vi "Interpolation_Solver.vi"(2 "Points Between":i32=10 min=0 step=1, 3 "Type of Interpolation":T2(ring), 4 "Data":dbl[][](array[numeric])=[[0.0, 1.0], [1.0, 2.700000047683716], [2.0, 7.400000095367432], [3.0, 150.0], [4.0, 80.0], [5.0, 220.0]] format="%.2f") -> (0 "Interpolated Data":dbl[](array[numeric])=[0.0, 0.09090909090909091, 0.18181818181818182, 0.2727272727272727, 0.36363636363636365, 0.45454545454545453, 0.5454545454545454, 0.6363636363636364, 0.7272727272727273, 0.8181818181818182, 0.9090909090909091, 1.0, 1.0909090909090908, 1.1818181818181819, 1.2727272727272727, 1.3636363636363635, 1.4545454545454546, 1.5454545454545454, 1.6363636363636365, 1.7272727272727273, 1.8181818181818181, 1.9090909090909092, 2.0, 2.090909090909091, 2.1818181818181817, 2.272727272727273, 2.3636363636363638, 2.4545454545454546, 2.5454545454545454, 2.6363636363636362, 2.727272727272727, 2.8181818181818183, 2.909090909090909, 3.0, 3.090909090909091, 3.1818181818181817, 3.272727272727273, 3.3636363636363638, 3.4545454545454546, 3.5454545454545454, 3.6363636363636362, 3.727272727272727, 3.8181818181818183, 3.909090909090909, 4.0, 4.090909090909091, 4.181818181818182, 4.2727272727272725, 4.363636363636363, 4.454545454545454, 4.545454545454546, 4.636363636363637, 4.7272727272727275, 4.818181818181818, 4.909090909090909, 5.0] format="%.2f", 1 "Interpolated X Axis":dbl[](array[numeric])=[0.0, 0.16666666666666666, 0.3333333333333333, 0.5, 0.6666666666666666, 0.8333333333333334, 1.0, 1.1666666666666667, 1.3333333333333333, 1.5, 1.6666666666666667, 1.8333333333333333, 2.0, 2.1666666666666665, 2.3333333333333335, 2.5, 2.6666666666666665, 2.8333333333333335, 3.0, 3.1666666666666665, 3.3333333333333335, 3.5, 3.6666666666666665, 3.8333333333333335, 4.0, 4.166666666666667, 4.333333333333333, 4.5, 4.666666666666667, 4.833333333333333, 5.0, 5.166666666666667, 5.333333333333333, 5.5, 5.666666666666667, 5.833333333333333, 6.0, 6.166666666666667, 6.333333333333333, 6.5, 6.666666666666667, 6.833333333333333, 7.0, 7.166666666666667, 7.333333333333333, 7.5, 7.666666666666667, 7.833333333333333, 8.0, 8.166666666666666, 8.333333333333334, 8.5, 8.666666666666666, 8.833333333333334, 9.0, 9.166666666666666, 9.333333333333334, 9.5, 9.666666666666666, 9.833333333333334, 10.0, 10.166666666666666, 10.333333333333334, 10.5, 10.666666666666666, 10.833333333333334, 11.0, 11.166666666666666, 11.333333333333334, 11.5, 11.666666666666666, 11.833333333333334, 12.0, 12.166666666666666, 12.333333333333334, 12.5, 12.666666666666666, 12.833333333333334, 13.0, 13.166666666666666, 13.333333333333334, 13.5, 13.666666666666666, 13.833333333333334, 14.0, 14.166666666666666, 14.333333333333334, 14.5, 14.666666666666666, 14.833333333333334, 15.0, 15.166666666666666, 15.333333333333334, 15.5, 15.666666666666666, 15.833333333333334, 16.0, 16.166666666666668, 16.333333333333332, 16.5, 16.666666666666668, 16.833333333333332, 17.0, 17.166666666666668, 17.333333333333332, 17.5, 17.666666666666668, 17.833333333333332, 18.0, 18.166666666666668, 18.333333333333332, 18.5, 18.666666666666668, 18.833333333333332, 19.0, 19.166666666666668, 19.333333333333332, 19.5, 19.666666666666668, 19.833333333333332, 20.0, 20.166666666666668, 20.333333333333332, 20.5, 20.666666666666668, 20.833333333333332, 21.0, 21.166666666666668, 21.333333333333332, 21.5, 21.666666666666668, 21.833333333333332, 22.0, 22.166666666666668, 22.333333333333332, 22.5, 22.666666666666668, 22.833333333333332, 23.0, 23.166666666666668, 23.333333333333332, 23.5, 23.666666666666668, 23.833333333333332, 24.0, 24.166666666666668, 24.333333333333332, 24.5, 24.666666666666668, 24.833333333333332, 25.0, 25.166666666666668, 25.333333333333332, 25.5, 25.666666666666668, 25.833333333333332, 26.0, 26.166666666666668, 26.333333333333332, 26.5, 26.666666666666668, 26.833333333333332, 27.0, 27.166666666666668, 27.333333333333332, 27.5, 27.666666666666668, 27.833333333333332, 28.0, 28.166666666666668, 28.333333333333332, 28.5, 28.666666666666668, 28.833333333333332, 29.0, 29.166666666666668, 29.333333333333332, 29.5, 29.666666666666668, 29.833333333333332, 30.0, 30.166666666666668, 30.333333333333332, 30.5, 30.666666666666668, 30.833333333333332, 31.0, 31.166666666666668, 31.333333333333332, 31.5, 31.666666666666668, 31.833333333333332, 32.0, 32.166666666666664, 32.333333333333336, 32.5, 32.666666666666664, 32.833333333333336, 33.0, 33.166666666666664, 33.333333333333336, 33.5, 33.666666666666664, 33.833333333333336, 34.0, 34.166666666666664, 34.333333333333336, 34.5, 34.666666666666664, 34.833333333333336, 35.0, 35.166666666666664, 35.333333333333336, 35.5, 35.666666666666664, 35.833333333333336, 36.0, 36.166666666666664, 36.333333333333336, 36.5, 36.666666666666664, 36.833333333333336, 37.0, 37.166666666666664, 37.333333333333336, 37.5, 37.666666666666664, 37.833333333333336, 38.0, 38.166666666666664, 38.333333333333336, 38.5, 38.666666666666664, 38.833333333333336, 39.0, 39.166666666666664, 39.333333333333336, 39.5, 39.666666666666664, 39.833333333333336, 40.0, 40.166666666666664, 40.333333333333336, 40.5, 40.666666666666664, 40.833333333333336, 41.0, 41.166666666666664, 41.333333333333336, 41.5, 41.666666666666664, 41.833333333333336, 42.0, 42.166666666666664, 42.333333333333336, 42.5, 42.666666666666664, 42.833333333333336, 43.0, 43.166666666666664, 43.333333333333336, 43.5, 43.666666666666664, 43.833333333333336, 44.0, 44.166666666666664, 44.333333333333336, 44.5, 44.666666666666664, 44.833333333333336, 45.0, 45.166666666666664, 45.333333333333336, 45.5, 45.666666666666664, 45.833333333333336, 46.0, 46.166666666666664, 46.333333333333336, 46.5, 46.666666666666664, 46.833333333333336, 47.0, 47.166666666666664, 47.333333333333336, 47.5, 47.666666666666664, 47.833333333333336, 48.0, 48.166666666666664, 48.333333333333336, 48.5, 48.666666666666664, 48.833333333333336, 49.0, 49.166666666666664, 49.333333333333336, 49.5, 49.666666666666664, 49.833333333333336, 50.0, 50.166666666666664, 50.333333333333336, 50.5, 50.666666666666664, 50.833333333333336, 51.0, 51.166666666666664, 51.333333333333336, 51.5, 51.666666666666664, 51.833333333333336, 52.0, 52.166666666666664, 52.333333333333336, 52.5, 52.666666666666664, 52.833333333333336, 53.0, 53.166666666666664, 53.333333333333336, 53.5, 53.666666666666664, 53.833333333333336, 54.0, 54.166666666666664, 54.333333333333336, 54.5, 54.666666666666664, 54.833333333333336, 55.0, 55.166666666666664, 55.333333333333336, 55.5, 55.666666666666664, 55.833333333333336, 56.0, 56.166666666666664, 56.333333333333336, 56.5, 56.666666666666664, 56.833333333333336, 57.0, 57.166666666666664, 57.333333333333336, 57.5, 57.666666666666664, 57.833333333333336, 58.0, 58.166666666666664, 58.333333333333336, 58.5, 58.666666666666664, 58.833333333333336, 59.0, 59.166666666666664, 59.333333333333336, 59.5, 59.666666666666664, 59.833333333333336, 60.0, 60.166666666666664, 60.333333333333336, 60.5, 60.666666666666664, 60.833333333333336, 61.0, 61.166666666666664, 61.333333333333336, 61.5, 61.666666666666664, 61.833333333333336, 62.0, 62.166666666666664, 62.333333333333336, 62.5, 62.666666666666664, 62.833333333333336, 63.0, 63.166666666666664, 63.333333333333336, 63.5, 63.666666666666664, 63.833333333333336, 64.0, 64.16666666666667, 64.33333333333333, 64.5, 64.66666666666667, 64.83333333333333, 65.0, 65.16666666666667, 65.33333333333333, 65.5, 65.66666666666667, 65.83333333333333, 66.0, 66.16666666666667, 66.33333333333333, 66.5, 66.66666666666667, 66.83333333333333, 67.0, 67.16666666666667, 67.33333333333333, 67.5, 67.66666666666667, 67.83333333333333, 68.0, 68.16666666666667, 68.33333333333333, 68.5, 68.66666666666667, 68.83333333333333, 69.0, 69.16666666666667, 69.33333333333333, 69.5, 69.66666666666667, 69.83333333333333, 70.0, 70.16666666666667, 70.33333333333333, 70.5, 70.66666666666667, 70.83333333333333, 71.0, 71.16666666666667, 71.33333333333333, 71.5, 71.66666666666667, 71.83333333333333, 72.0, 72.16666666666667, 72.33333333333333, 72.5, 72.66666666666667, 72.83333333333333, 73.0, 73.16666666666667, 73.33333333333333, 73.5, 73.66666666666667, 73.83333333333333, 74.0, 74.16666666666667, 74.33333333333333, 74.5, 74.66666666666667, 74.83333333333333, 75.0, 75.16666666666667, 75.33333333333333, 75.5, 75.66666666666667, 75.83333333333333, 76.0, 76.16666666666667, 76.33333333333333, 76.5, 76.66666666666667, 76.83333333333333, 77.0, 77.16666666666667, 77.33333333333333, 77.5, 77.66666666666667, 77.83333333333333, 78.0, 78.16666666666667, 78.33333333333333, 78.5, 78.66666666666667, 78.83333333333333, 79.0, 79.16666666666667, 79.33333333333333, 79.5, 79.66666666666667, 79.83333333333333, 80.0, 80.16666666666667, 80.33333333333333, 80.5, 80.66666666666667, 80.83333333333333, 81.0, 81.16666666666667, 81.33333333333333, 81.5, 81.66666666666667, 81.83333333333333, 82.0, 82.16666666666667, 82.33333333333333, 82.5, 82.66666666666667, 82.83333333333333, 83.0, 83.16666666666667, 83.33333333333333, 83.5, 83.66666666666667, 83.83333333333333, 84.0, 84.16666666666667, 84.33333333333333, 84.5, 84.66666666666667, 84.83333333333333, 85.0, 85.16666666666667, 85.33333333333333, 85.5, 85.66666666666667, 85.83333333333333, 86.0, 86.16666666666667, 86.33333333333333, 86.5, 86.66666666666667, 86.83333333333333, 87.0, 87.16666666666667, 87.33333333333333, 87.5, 87.66666666666667, 87.83333333333333, 88.0, 88.16666666666667, 88.33333333333333, 88.5, 88.66666666666667, 88.83333333333333, 89.0, 89.16666666666667, 89.33333333333333, 89.5, 89.66666666666667, 89.83333333333333, 90.0, 90.16666666666667, 90.33333333333333, 90.5, 90.66666666666667, 90.83333333333333, 91.0, 91.16666666666667, 91.33333333333333, 91.5, 91.66666666666667, 91.83333333333333, 92.0, 92.16666666666667, 92.33333333333333, 92.5, 92.66666666666667, 92.83333333333333, 93.0, 93.16666666666667, 93.33333333333333, 93.5, 93.66666666666667, 93.83333333333333, 94.0, 94.16666666666667, 94.33333333333333, 94.5, 94.66666666666667, 94.83333333333333, 95.0, 95.16666666666667, 95.33333333333333, 95.5, 95.66666666666667, 95.83333333333333, 96.0, 96.16666666666667, 96.33333333333333, 96.5, 96.66666666666667, 96.83333333333333, 97.0, 97.16666666666667, 97.33333333333333, 97.5, 97.66666666666667, 97.83333333333333, 98.0, 98.16666666666667, 98.33333333333333, 98.5, 98.66666666666667, 98.83333333333333, 99.0, 99.16666666666667, 99.33333333333333, 99.5, 99.66666666666667, 99.83333333333333, 100.0, 100.16666666666667, 100.33333333333333, 100.5, 100.66666666666667, 100.83333333333333, 101.0, 101.16666666666667, 101.33333333333333, 101.5, 101.66666666666667, 101.83333333333333, 102.0, 102.16666666666667, 102.33333333333333] format="%.4f")   [LabVIEW 2019]
doc: "This example demonstrates the use of various interpolation VIs including:\n Linear Interpolation\n Polynomial Interpolation\n Spline Interpolation\n Rational Interpolation"
uses:
  <vilib>/Utility/file.llb/Read From Spreadsheet File (DBL).vi
  <vilib>/Utility/file.llb/Write To Spreadsheet File (DBL).vi
  <vilib>/Analysis/NI_AALPro.lvlib
panel:
  in  "data selector":T1(ring)
  out "Raw Data and Interpolated Data":cluster{dbl[], "Best Exponential Fit":dbl[]}[](graph)=[{[0.0, 1.0, 2.0, 3.0, 4.0, 5.0], "Best Exponential Fit"=[1.0, 2.700000047683716, 7.400000095367432, 150.0, 80.0, 220.0]}, {[0.0, 0.09090909090909091, 0.18181818181818182, 0.2727272727272727, 0.36363636363636365, 0.45454545454545453, 0.5454545454545454, 0.6363636363636364, 0.7272727272727273, 0.8181818181818182, 0.9090909090909091, 1.0, 1.0909090909090908, 1.1818181818181819, 1.2727272727272727, 1.3636363636363635, 1.4545454545454546, 1.5454545454545454, 1.6363636363636365, 1.7272727272727273, 1.8181818181818181, 1.9090909090909092, 2.0, 2.090909090909091, 2.1818181818181817, 2.272727272727273, 2.3636363636363638, 2.4545454545454546, 2.5454545454545454, 2.6363636363636362, 2.727272727272727, 2.8181818181818183, 2.909090909090909, 3.0, 3.090909090909091, 3.1818181818181817, 3.272727272727273, 3.3636363636363638, 3.4545454545454546, 3.5454545454545454, 3.6363636363636362, 3.727272727272727, 3.8181818181818183, 3.909090909090909, 4.0, 4.090909090909091, 4.181818181818182, 4.2727272727272725, 4.363636363636363, 4.454545454545454, 4.545454545454546, 4.636363636363637, 4.7272727272727275, 4.818181818181818, 4.909090909090909, 5.0], "Best Exponential Fit"=[1.0, 1.2152761356490307, 1.780613923204889, 2.575277433580718, 3.4785307376896637, 4.36963790644487, 5.127863010759482, 5.632470121546648, 5.762723309719508, 5.397886646191209, 4.417224201874898, 2.700000047683716, 0.20566834793003874, -2.785556359476875, -5.91326944322851, -8.817066272016389, -11.136542214532014, -12.511292639466877, -12.580912915512496, -10.98499841136037, -7.363144495702005, -1.3549465372288942, 7.400000095367432, 19.083237862020354, 33.16086053716275, 48.92009972385246, 65.64818702514707, 82.6323540441044, 99.15983238378223, 114.5178536472383, 127.99364943753035, 138.8744513577162, 146.44749101085347, 150.0, 149.08978031624378, 144.3569155027938, 136.71205949088926, 127.06586621176949, 116.32898959667368, 105.41208357684113, 95.225802083511, 86.68079904792259, 80.68772840131508, 78.15724407492783, 80.0, 86.80407219935121, 97.86722506212251, 112.16464506903529, 128.671518700811, 146.36303243817096, 164.21437276183684, 181.2007261525296, 196.29727909097096, 208.47921805788215, 216.72172953398473, 220.0]}]
  # "Data"
  # "x"
  # "y"
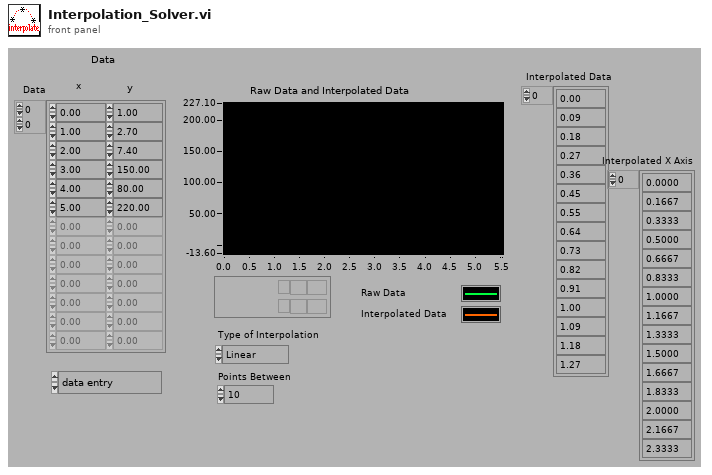
[diagram p1: front panel]
types:
  T1 = enum16{"data entry", "read from file", "write to file"}
  T2 = enum16{"Linear", "Polynomial", "Spline", "Rational"}
  T3 = cluster{"Type of Interpolation":enum16{"Linear", "Polynomial", "Spline", "Rational"}, "Points Between":i32}
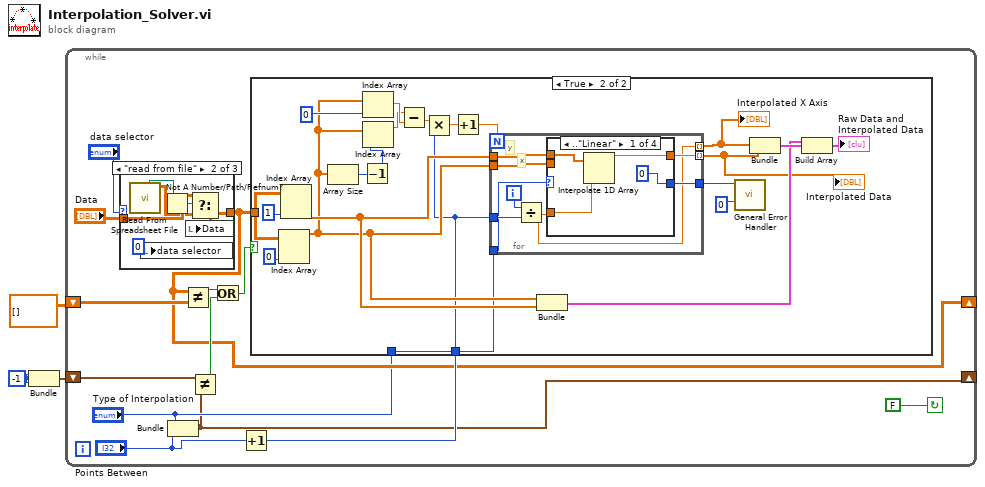
[diagram p0: block diagram]
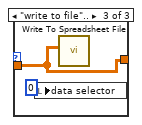
[diagram p3: hidden frame]
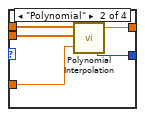
[diagram p5: hidden frame]
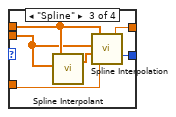
[diagram p6: hidden frame]
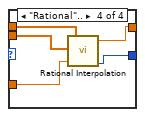
[diagram p7: hidden frame]
diagram:
  w1 = -1
  n1 = Bundle(w1, w1) -> (w2:cluster{i32, i32})  [unwired: 1 in]
  n2 = while {
    shift-left: w2 -> [w6]
    shift-right: [w5] -> _
    shift-left: dbl[][] [] -> [w16]
    shift-right: [w9] -> _
    stop <- FALSE continue-if-true
    n3 = case shown="\"read from file\"" "data selector" {
      tunnel: [w17 w19 w25] -> w9
      tunnel: "Data" -> [w17 w21 w25]
      frame .."data entry" {
      }
      frame "read from file" {
        n4 = call-poly <vilib>:"Read From Spreadsheet File.vi"() -> ("all rows"=w20:dbl[][], "new file path (Not A Path if cancelled)"=w23:path)  [unwired: 7 in, 3 out]
        n5 = local write "data selector"(0) -> ()
        n6 = Not A Number/Path/Refnum?(number/path/refnum=w23) -> (NaN/Path/Refnum?=w22:bool)
        n7 = Select(t=w21, s=w22, f=w20) -> (s? t:f=w19:dbl[][])
        n8 = local write "Data"(w19) -> ()
      }
      frame "write to file".. {
        n9 = local write "data selector"(0) -> ()
        n10 = call-poly <vilib>:"Write To Spreadsheet File.vi"("2D data"=w25) -> ()  [unwired: 7 in, 1 out]
      }
    }
    n11 = Bundle("Type of Interpolation"="Type of Interpolation", "Points Between"="Points Between") -> (w5:T3)  [unwired: 1 in]
    n12 = Not Equal?(x=w9, y=w16) -> (x != y?=w12:bool)
    n13 = Not Equal?(x=w6, y=w5) -> (x != y?=w11:bool)
    n14 = Or(x=w12, y=w11) -> (x .or. y?=w10:bool)
    n15 = Increment(x="Points Between") -> (x+1=w13:i32)
    n16 = case shown="True" w10 {
      tunnel: w9 -> [_ w40]
      tunnel: "Type of Interpolation" -> [_ w34]
      tunnel: w13 -> [_ w27]
      frame False {
      }
      frame True {
        n17 = Index Array(array=w40, index (col)=0) -> (element=w36:dbl[])  [unwired: 1 in]
        n18 = Index Array(array=w40, index (col)=1) -> (element=w37:dbl[])  [unwired: 1 in]
        n19 = Array Size(array=w36) -> (size(s)=w39:i32)
        n20 = Decrement(x=w39) -> (x-1=w35:i32)
        n21 = Index Array(array=w36, index=0) -> (element=w30:dbl)
        n22 = Index Array(array=w36, index=w35) -> (element=w29:dbl)
        n23 = Subtract(x=w29, y=w30) -> (x-y=w32:dbl)
        n24 = Multiply(x=w32, y=w27) -> (x*y=w33:dbl)
        n25 = Increment(x=w33) -> (x+1=w31:dbl)
        n26 = for {
          N: w31 -> [_]
          tunnel: w37 -> [w55]
          tunnel: w36 -> [w54]
          tunnel: [w53] -> w47
          tunnel: w34 -> [w48]
          tunnel: w27 -> [w51]
          tunnel: [w50] -> w28 mode=indexing
          tunnel: [w49] -> w26 mode=indexing
          i -> [w52]
          # "x"
          # "y"
          n27 = Divide(x=w52, y=w51) -> (x/y=w49:dbl)
          n28 = case shown="..\"Linear\"" w48 {
            tunnel: w49 -> [w58 w64 w67 w71]
            tunnel: [w57 w63 w65 w73] -> w50
            tunnel: [0 w62 w66 w72] -> w53
            tunnel: w54 -> [_ w61 w68 w74]
            tunnel: w55 -> [w59 w60 w70 w75]
            frame .."Linear" {
              n29 = Interpolate 1D Array(1:w58, 2:w59) -> (0:w57:dbl)
            }
            frame "Polynomial" {
              n30 = call <vilib>:"Polynomial Interpolation.vi"("x value"=w64, "X"=w61, "Y"=w60) -> ("error"=w62:i32, "interpolation value"=w63:dbl)  [unwired: 1 out]
            }
            frame "Spline" {
              n31 = call <vilib>:"Spline Interpolant.vi"("X"=w68, "Y"=w70) -> ("Interpolant"=w69:dbl[])  [unwired: 2 in, 1 out]
              n32 = call <vilib>:"Spline Interpolation.vi"("x value"=w67, "Interpolant"=w69, "X"=w68, "Y"=w70) -> ("error"=w66:i32, "interpolation value"=w65:dbl)
            }
            frame "Rational".. {
              n33 = call <vilib>:"Rational Interpolation.vi"("x value"=w71, "X"=w74, "Y"=w75) -> ("error"=w72:i32, "interpolation value"=w73:dbl)  [unwired: 1 out]
            }
          }
        }
        "Interpolated Data" <- w28
        "Interpolated X Axis" <- w26
        n34 = Bundle("Data"=w36, "Data"=w37) -> (w42:cluster{"Data":dbl[], "Data":dbl[]})  [unwired: 1 in]
        n35 = call <vilib>:"General Error Handler.vi"("[error code] (0)"=w47, "type of dialog (OK msg:1)"=0) -> ()  [unwired: 9 in, 5 out]
        n36 = Bundle(w26, w28) -> (w46:cluster{dbl[], dbl[]})  [unwired: 1 in]
        n37 = Build Array(w42, w46) -> (→"Raw Data and Interpolated Data":cluster{"Data":dbl[], "Data":dbl[]}[])
      }
    }
  }
